vi "Create Table Refnum.vi"(5 "Table properties":T1={"Table position"=1, "SpacingBefore (points)"=12.0, "SpacingAfter (points)"=12.0} {"Table position" items=["LEFT", "CENTER", "RIGHT"]}, 6 "error in (no error)":errorcluster, 7 "columnWidth [ ]":sgl[](array[numeric])=[0.0], 8 "numColumns":i32, 9 "PDF Report":T23(xcontrol)) -> (0 "error out":errorcluster, 1 "columnWidth (points)":sgl[](array[numeric]), 2 "PdfP Table ref":refnum<k24>, 3 "PDF Report duplicate":T23(xcontrol))   [LabVIEW 2012]
doc: "<B>ENGLISH</B>\nCreates a table with the given <B>numColumns</B> and the given <B>columnWidth [ ]</B>.\n\n<B>FRANÇAIS</B>\nCréation d'un tableau avec pour nombre de colonnes <B>numColumns</B> et dont les largeurs sont spécifiées par <B>columnWidth [ ]</B>.\n\nVersion 1.0\nDeveloped by Jean-Marc Simard\nCopyright © 2010, Exaprom Inc.\nAll rights reserved.\nLicense: BSD\n\nWith iTextSharp 4.1.6 (http://itextsharp.sourceforge.net)\nunder Mozilla Public License Version 1.1\n(http://www.mozilla.org/MPL/MPL-1.1.html)"
uses:
  Controls/PDF Report Xcontrol/PDF Report.xctl
  C:/Users/MaxCorp/Documents/TopPerm - Base/DLL/itextsharp.dll
  DLL/itextsharp.dll
  Controls/Table properties.ctl
  Controls/Table position.ctl
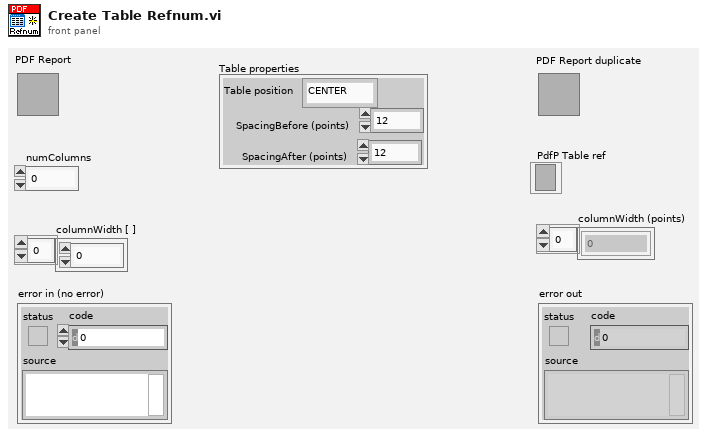
[diagram p1: front panel]
types:
  T1 = typedef "Table properties.ctl" = cluster{"Table position":T2, "SpacingBefore (points)":sgl, "SpacingAfter (points)":sgl}
  T2 = typedef "Table position.ctl" = i32
  T3 = typedef "Font cluster.ctl" = cluster{"Name":string, "Size":T4, "Color":T5, "Style":cluster{"Bold":bool, "Italic":bool, "Underline":bool, "Strikeout":bool}}
  T4 = typedef "Font size.ctl" = sgl
  T5 = typedef "Font color.ctl" = u32
  T6 = typedef "Unit.ctl" = enum16{"inch", "mm"}
  T7 = typedef "Paragraphe cluster.ctl" = cluster{" Aligment":T8, "Line spacing":T9}
  T8 = typedef "Texte alignement.ctl" = enum16{"Select", "CENTER", "JUSTIFY", "LEFT", "RIGHT"}
  T9 = typedef "Line spacing.ctl" = enum16{"Select", "1.0", "1.5", "2.0"}
  T10 = typedef "Page dimensions.ctl" = cluster{"Start at page":i32, "Orientation":T11, "widht":sgl, "height":sgl, "Margin left":sgl, "Margin right":sgl, "Margin top":sgl, "Margin bottom":sgl}
  T11 = typedef "Page Orientation.ctl" = enum16{"Portrait", "Landscape"}
  T12 = typedef "Image or Table Caption.ctl" = cluster{"Caption":string, "Separator":string, "Position":enum16{"Above", "Below"}}
  T13 = typedef "Header Footer [ ].ctl" = T14[]
  T14 = typedef "Header Footer cluster.ctl" = cluster{"Start page":i32, "Type":T15, "Alignment":T16, "Vertical Alignement":T17, "Image (%)":sgl, "Page #":T18, "Text":string, "Path":string, "Font":T3, "Font refnum":refnum<k24>, "Line":cluster{"Line":T19, "Thickness (points)":sgl, "Colour":T5}}
  T15 = typedef "Header Footer Type.ctl" = enum16{"Select", "Text", "Text + hyperlink", "Page number", "Image", "Image + hyperlink"}
  T16 = typedef "Header footer horiz alignment.ctl" = enum16{"Left", "Center", "Right"}
  T17 = typedef "Cell Vertical alignment.ctl" = enum16{"TOP", "MIDDLE", "BOTTOM"}
  T18 = typedef "Page number.ctl" = cluster{"Text 1":string, "Text 2":string, "Text 3":string}
  T19 = typedef "Header Footer Line.ctl" = enum16{"No line", "Horizontal line"}
  T20 = typedef "Watermark cluster2.ctl" = cluster{"Show? (F)":bool, "Type":enum16{"Image", "Text"}, "Opacity (%)":sgl, "Rotate(°)":sgl, "Position":cluster{"Position":T21, "X":sgl, "Y":sgl}, "Image path":path, "Scaled(%)":sgl, "Image refnum":refnum<k24>, "Text":string, "Font":cluster{"Name":string, "Size":T4, "Color":T5}, "Font refnum":refnum<k24>, "Alignment":T16, "Automatic":bool}
  T21 = typedef "Watermark Position.ctl" = enum16{"Absolute", "Center (page)", "Center (text section)"}
  T22 = typedef "System Fonts.ctl" = cluster{"Font name [ ]":string[], "Font and file names [ ]":cluster{"Font name":string, "File name":string}[]}
  T23 = cluster{"Document":refnum<k24>, "Writer":refnum<k24>, "Default Font":refnum<k24>, "Default Font cluster":T3, "Path":path, "Unit (default = mm)":T6, "Paragraphe cluster":T7, "Pages dimensions [ ]":T10[], "Captions":cluster{"Image":T12, "Image counter":u16, "Table":T12, "Table counter":u16, "Font":T3}, "Header":T13, "Footer":T13, "Watermark ":T20, "Actual VI name":string, "System Fonts":T22}
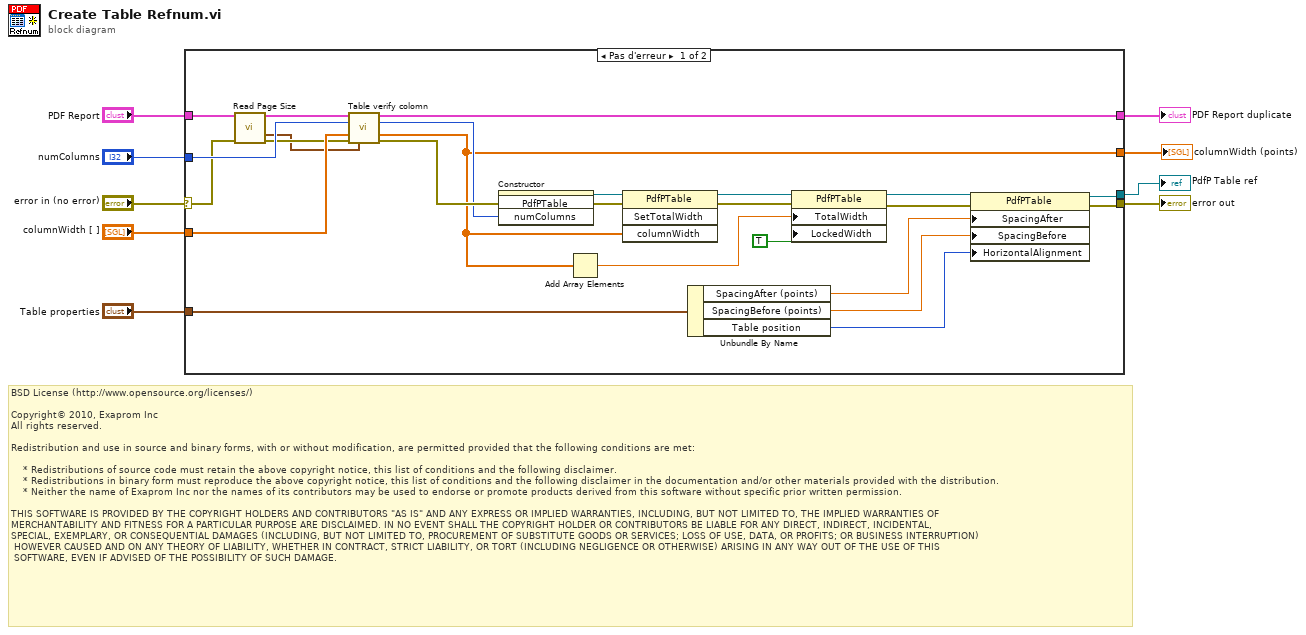
[diagram p0: block diagram]
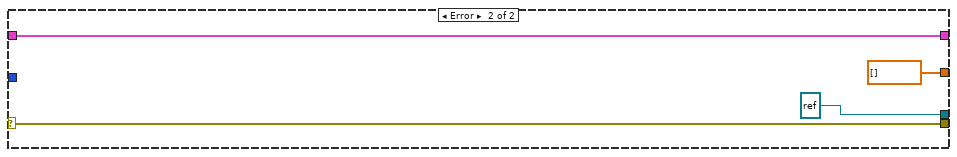
[diagram p2: hidden frame]
diagram:
  # "BSD License (http://www.opensource.org/licenses/)\n\nCopyright© 2010, Exaprom Inc\nAll rights reserved.\n\nRedistribution and use in source and binary forms, with or without modification, are permitted provided that the following conditions are met:\n\n    * Redistributions of source code must retain the above copyright notice, this list of conditions and the following disclaimer.\n    * Redistributions in binary form must reproduce the above copyright notice, this list of conditions and the following disclaimer in the documentation and/or other materials provided with the distribution.\n    * Neither the name of Exaprom Inc nor the names of its contributors may be used to endorse or promote products derived from this software without specific prior written permission.\n\nTHIS SOFTWARE IS PROVIDED BY THE COPYRIGHT HOLDERS AND CONTRIBUTORS \"AS IS\" AND ANY EXPRESS OR IMPLIED WARRANTIES, INCLUDING, BUT NOT LIMITED TO, THE IMPLIED WARRANTIES OF \nMERCHANTABILITY AND FITNESS FOR A PARTICULAR PURPOSE ARE DISCLAIMED. IN NO EVENT SHALL THE COPYRIGHT HOLDER OR CONTRIBUTORS BE LIABLE FOR ANY DIRECT, INDIRECT, INCIDENTAL,\nSPECIAL, EXEMPLARY, OR CONSEQUENTIAL DAMAGES (INCLUDING, BUT NOT LIMITED TO, PROCUREMENT OF SUBSTITUTE GOODS OR SERVICES; LOSS OF USE, DATA, OR PROFITS; OR BUSINESS INTERRUPTION)\n HOWEVER CAUSED AND ON ANY THEORY OF LIABILITY, WHETHER IN CONTRACT, STRICT LIABILITY, OR TORT (INCLUDING NEGLIGENCE OR OTHERWISE) ARISING IN ANY WAY OUT OF THE USE OF THIS\n SOFTWARE, EVEN IF ADVISED OF THE POSSIBILITY OF SUCH DAMAGE."
  n1 = case shown="Pas d'erreur" "error in (no error)" {
    selector: "error in (no error)" -> [w10 w38]
    tunnel: "numColumns" -> [w25 _]
    tunnel: "columnWidth [ ]" -> [w26 _]
    tunnel: [w15 w38] -> w6
    tunnel: [w16 refnum<k24> refnum ("new reference")] -> w5
    tunnel: [w24 w36] -> w4
    tunnel: "PDF Report" -> [w22 w36]
    tunnel: "Table properties" -> [w17 _]
    tunnel: [w11 sgl[] [] ("columnWidth (points)")] -> w1
    frame No Error {
      n2 = call "Read Page Size.vi"("PDF Report"=w22, "error in (no error)"=w10) -> ("PDF Report duplicate"=w23:T23, "Page (points)"=w20:T10, "error out"=w21:errorcluster)  [unwired: 11 out]
      n3 = call "Table verify colomn.vi"("PDF Report"=w23, "numColumns"=w25, "columnWidth"=w26, "error in (no error)"=w21, "Pages dimensions"=w20) -> ("PDF Report duplicate"=w24:T23, "numColumns duplicate"=w27:i32, "columnWidth (points)"=w11:sgl[], "error out"=w28:errorcluster)  [unwired: 7 out]
      n4 = constructor class="PdfPTable"(error in=w28, "numColumns"=w27) -> (reference out=w33:refnum<k24>, error out=w34:errorcluster)  [unwired: 2 in, 2 out]
      n5 = Add Array Elements(numeric array=w11) -> (sum=w29:sgl)
      n6 = invoke class="PdfPTable" method="SetTotalWidth"(reference=w33, error in=w34, "columnWidth"=w11) -> (reference out=w32:refnum<k24>, error out=w31:errorcluster)  [unwired: 1 in, 2 out]
      n7 = Unbundle By Name(w17) -> ("SpacingAfter (points)"=w14:sgl, "SpacingBefore (points)"=w13:sgl, "Table position"=w12:T2)
      n8 = property class="PdfPTable"(reference=w32, error in=w31, "TotalWidth"=w29, "LockedWidth"=TRUE) -> (reference out=w19:refnum<k24>, error out=w18:errorcluster)
      n9 = property class="PdfPTable"(reference=w19, error in=w18, "SpacingAfter"=w14, "SpacingBefore"=w13, "HorizontalAlignment"=w12) -> (reference out=w16:refnum<k24>, error out=w15:errorcluster)
    }
    frame Error {
    }
  }
  "error out" <- w6
  "PDF Report duplicate" <- w4
  "PdfP Table ref" <- w5
  "columnWidth (points)" <- w1
